vi "Wire Tag Terminals.vi"(6 "State":T1={"Worker Library Path"=path "", "Block Label"="", "Types"=[], "Selections"=[], "Icon"={"image type"=0, "image depth"=0, "image"=[], "mask"=[], "colors"=[], "Rectangle"={"left"=0, "top"=0, "right"=0, "bottom"=0}}, "Errors"={"Terminals"=[], "Generate"={"status"=FALSE, "code"=0, "source"=""}, "General"={"status"=FALSE, "code"=0, "source"=""}}, "Calculated Sizes"={"Block Width"=0, "Block Height"=0, "Half Width"=0, "Icon Top"=0, "Icon Bottom"=0, "Label Width"=0, "Half Label"=0, "Label Top"=0, "Text Width"=0, "Half Text"=0, "Text Height"=0, "Label Height"=0, "Expanded Width"=0, "Label Bottom"=0, "Expanded Top"=0, "Expanded Bottom"=0, "Expanded Height"=0, "Min Height"=0, "Max Height"=0}, "Special Terminal Indices"={"Action"=-1, "Init"=-1, "Tag"=-1, "State in"=-1, "State out"=-1, "Error"=-1}, "Terminals"=[]}, 8 "error in (no error)":errorcluster, 10 "Grouped Terms":T13, 11 "Refs In":T15) -> (0 "error out":errorcluster, 3 "Refs":T15)   [LabVIEW 2022 SP3, in "FlexBlocks Support.lvlib"]
uses:
  FlexBlocks Support.lvlib
  SM Refs.ctl
  Grouped Terms.ctl
  Terminal Group.ctl
  Type Descriptor.ctl
  Terminal Direction.ctl
  Value Mode.ctl
  Special Terminal.ctl
  Terminal State.ctl
  Flex Block/State.ctl
  <vilib>/picture/picture.llb/imagedata.ctl
  XNode Errors.ctl
  Calculated Sizes.ctl
  Special Terminal Indices.ctl
  Terminal Status.ctl
  Terminal Draw Style.ctl
  Flex Block/Flex Block.xnode
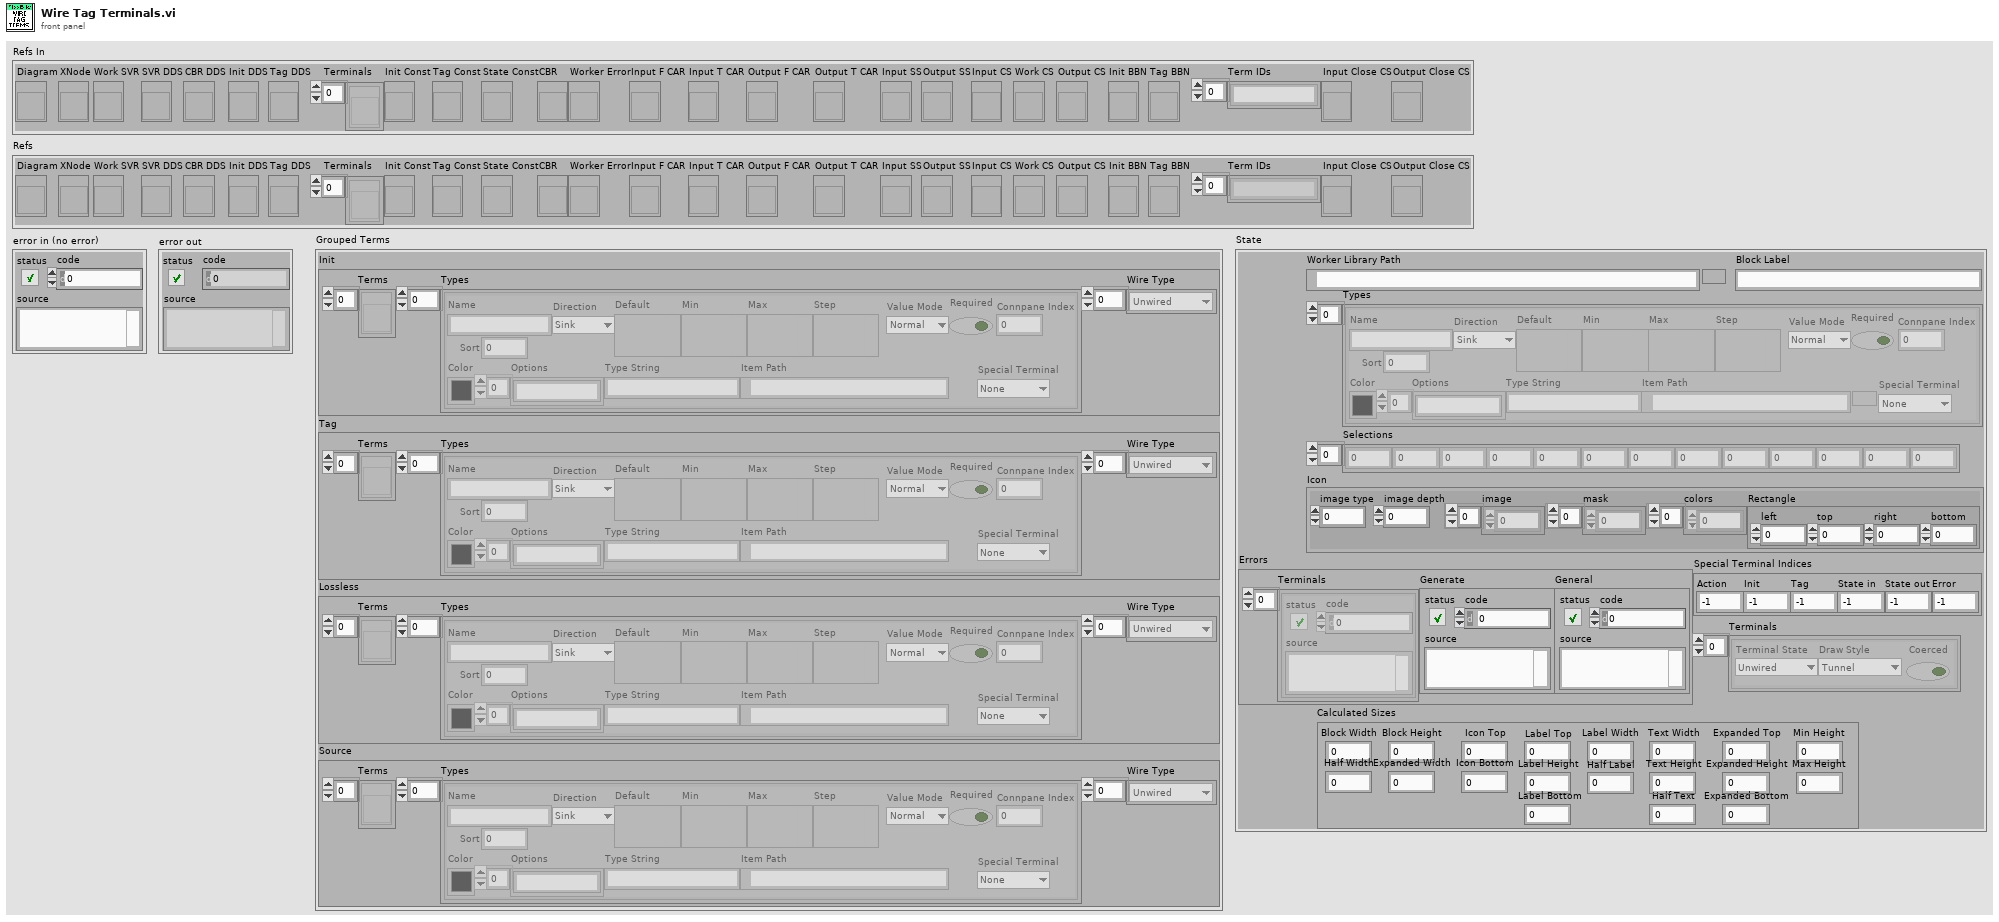
[diagram p1: front panel]
types:
  T1 = typedef "Flex Block.xnode/State.ctl" = cluster{"Worker Library Path":path, "Block Label":string, "Types":T2[], "Selections":i32[], "Icon":T6, "Errors":T7, "Calculated Sizes":T8, "Special Terminal Indices":T9, "Terminals":T10[]}
  T2 = typedef "FlexBlocks Support.lvlib/Type Descriptor.ctl" = cluster{"Name":string, "Direction":T3, "Default":variant, "Min":variant, "Max":variant, "Step":variant, "Value Mode":T4, "Color":u32, "Options":string[], "Type String":string, "Item Path":path, "Required":bool, "Connpane Index":i32, "Special Terminal":T5, "Sort":i32}
  T3 = typedef "FlexBlocks Support.lvlib/Terminal Direction.ctl" = enum16{"Sink", "Source"}
  T4 = typedef "FlexBlocks Support.lvlib/Value Mode.ctl" = enum16{"Normal", "Range", "Select"}
  T5 = typedef "FlexBlocks Support.lvlib/Special Terminal.ctl" = enum16{"None", "Action", "Init", "Tag", "State in", "State out", "Error"}
  T6 = typedef "imagedata.ctl" = cluster{"image type":i32, "image depth":i32, "image":u8[], "mask":u8[], "colors":u32[], "Rectangle":cluster{"left":i16, "top":i16, "right":i16, "bottom":i16}}
  T7 = typedef "FlexBlocks Support.lvlib/XNode Errors.ctl" = cluster{"Terminals":errorcluster[], "Generate":errorcluster, "General":errorcluster}
  T8 = typedef "FlexBlocks Support.lvlib/Calculated Sizes.ctl" = cluster{"Block Width":i32, "Block Height":i32, "Half Width":i32, "Icon Top":i32, "Icon Bottom":i32, "Label Width":i32, "Half Label":i32, "Label Top":i32, "Text Width":i32, "Half Text":i32, "Text Height":i32, "Label Height":i32, "Expanded Width":i32, "Label Bottom":i32, "Expanded Top":i32, "Expanded Bottom":i32, "Expanded Height":i32, "Min Height":i32, "Max Height":i32}
  T9 = typedef "FlexBlocks Support.lvlib/Special Terminal Indices.ctl" = cluster{"Action":i32, "Init":i32, "Tag":i32, "State in":i32, "State out":i32, "Error":i32}
  T10 = typedef "FlexBlocks Support.lvlib/Terminal Status.ctl" = cluster{"Terminal State":T11, "Draw Style":T12, "Coerced":bool}
  T11 = typedef "FlexBlocks Support.lvlib/Terminal State.ctl" = enum16{"Unwired", "BadType", "BadRef", "Channel", "Value", "Control Ref"}
  T12 = typedef "FlexBlocks Support.lvlib/Terminal Draw Style.ctl" = enum16{"Tunnel", "BadType", "BadRef", "Channel", "Value", "Control Ref"}
  T13 = typedef "FlexBlocks Support.lvlib/Grouped Terms.ctl" = cluster{"Init":T14, "Tag":T14, "Lossless":T14, "Source":T14}
  T14 = typedef "FlexBlocks Support.lvlib/Terminal Group.ctl" = cluster{"Terms":refnum<vi>[], "Types":T2[], "Wire Type":T11[]}
  T15 = typedef "FlexBlocks Support.lvlib/SM Refs.ctl" = cluster{"Diagram":refnum<vi>, "XNode":refnum<vi>, "Work SVR":refnum<vi>, "SVR DDS":refnum<vi>, "CBR DDS":refnum<vi>, "Init DDS":refnum<vi>, "Tag DDS":refnum<vi>, "Terminals":refnum<vi>[], "Init Const":refnum<vi>, "Tag Const":refnum<vi>, "State Const":refnum<vi>, "CBR":refnum<vi>, "Worker Error":refnum<vi>, "Input F CAR":refnum<vi>, "Input T CAR":refnum<vi>, "Output F CAR":refnum<vi>, "Output T CAR":refnum<vi>, "Input SS":refnum<vi>, "Output SS":refnum<vi>, "Input CS":refnum<vi>, "Work CS":refnum<vi>, "Output CS":refnum<vi>, "Init BBN":refnum<vi>, "Tag BBN":refnum<vi>, "Term IDs":string[], "Input Close CS":refnum<vi>, "Output Close CS":refnum<vi>}
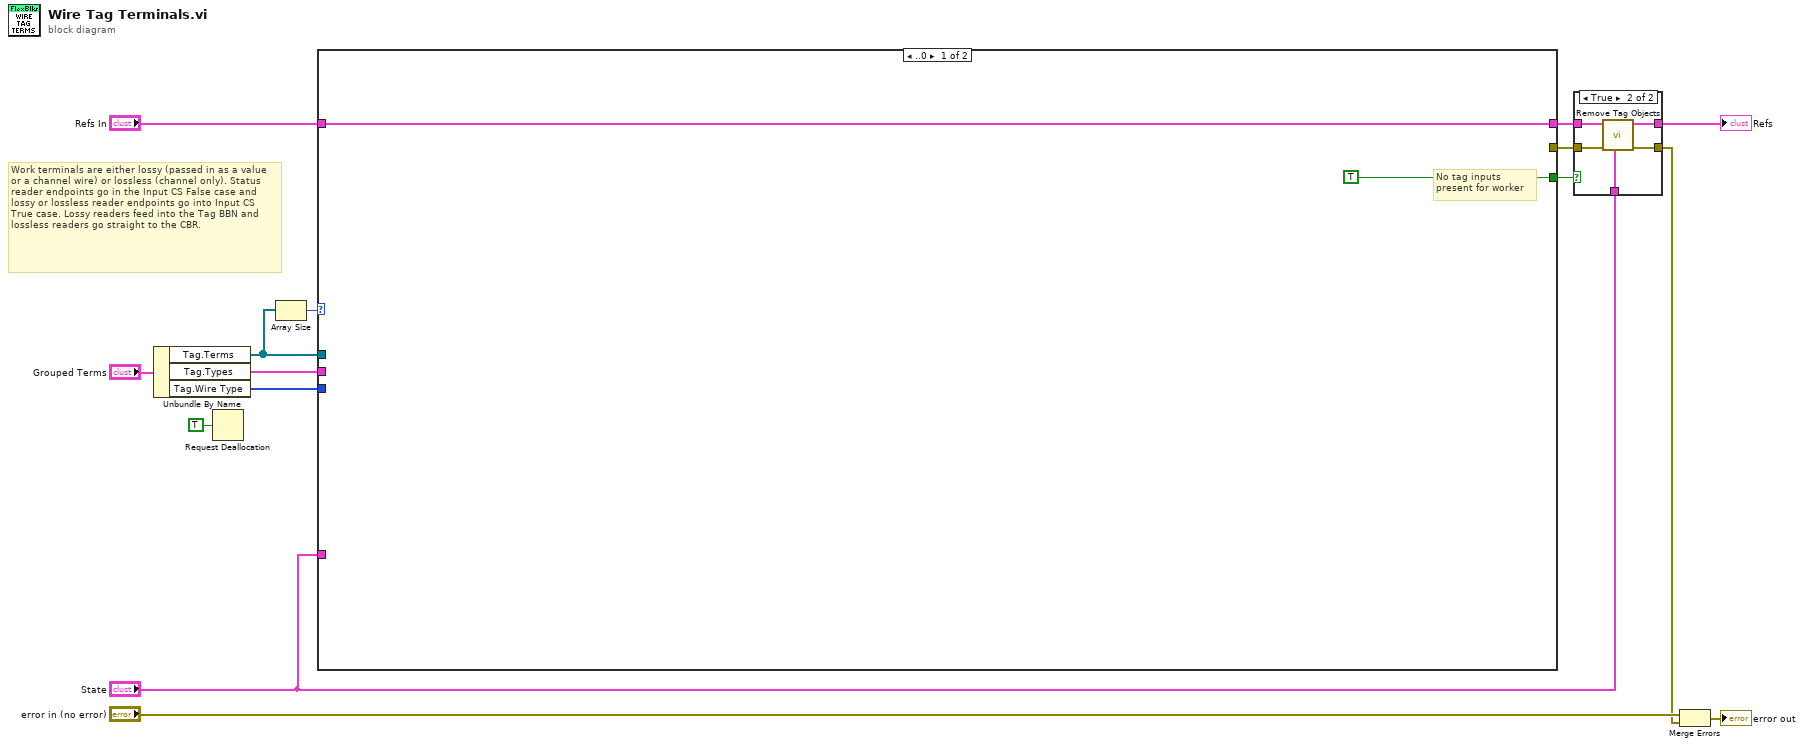
[diagram p0: block diagram]
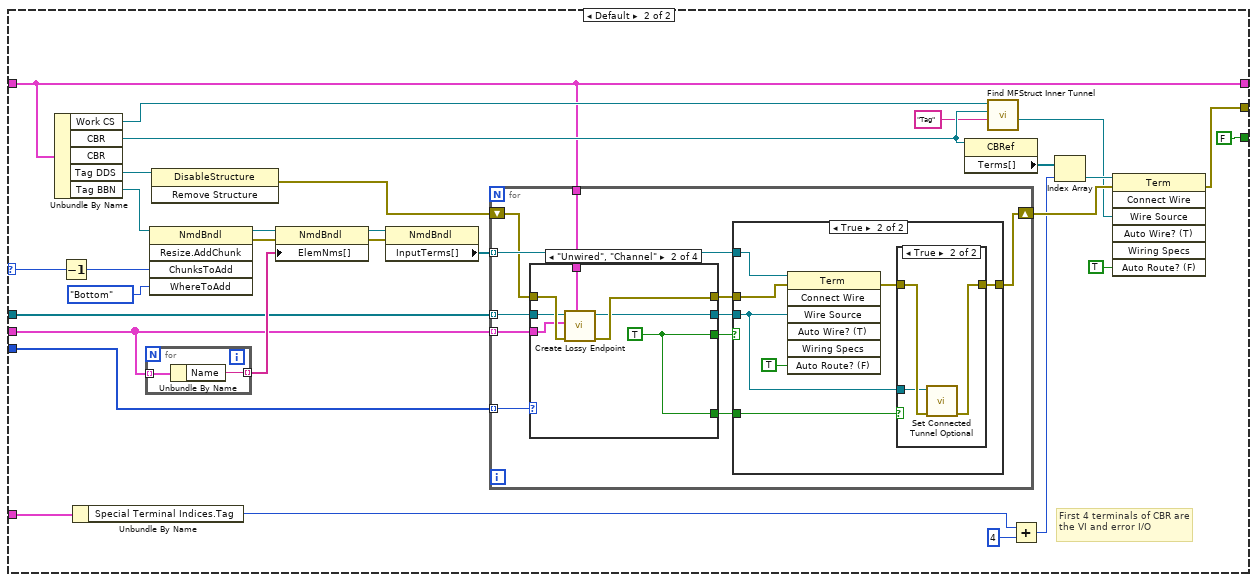
[diagram p2: hidden frame]
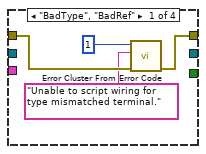
[diagram p3: hidden frame]
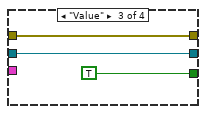
[diagram p4: hidden frame]
diagram:
  # "Work terminals are either lossy (passed in as a value or a channel wire) or lossless (channel only). Status reader endpoints go in the Input CS False case and lossy or lossless reader endpoints go into Input CS True case. Lossy readers feed into the Tag BBN and lossless readers go straight to the CBR."
  n1 = Unbundle By Name("Grouped Terms") -> ("Tag.Terms"=w13:refnum<vi>[], "Tag.Types"=w12:T2[], "Tag.Wire Type"=w3:T11[])
  n2 = Request Deallocation(TRUE ("flag")) -> ()
  n3 = Array Size(array=w13) -> (size(s)=w14:i32)
  n4 = case shown="..0" w14 {
    selector: w14 -> [_ w24]
    tunnel: w13 -> [_ w22]
    tunnel: w12 -> [_ w23]
    tunnel: "State" -> [_ w21]
    tunnel: "Refs In" -> [w17 w19]
    tunnel: [w17 w19] -> w10
    tunnel: [TRUE FALSE] -> w4
    tunnel: w3 -> [_ w20]
    tunnel: [_ w18] -> w1
    frame ..0 {
      # "No tag inputs present for worker"
    }
    frame Default {
      # "First 4 terminals of CBR are the VI and error I/O"
      n5 = Unbundle By Name(w19) -> ("Work CS"=w31:refnum<vi>, "CBR"=w30:refnum<vi>, "Tag DDS"=w44:refnum<vi>, "Tag BBN"=w43:refnum<vi>)  [unwired: 1 out]
      n6 = Decrement(x=w24) -> (x-1=w42:i32)
      n7 = Unbundle By Name(w21) -> ("Special Terminal Indices.Tag"=w33:i32)
      n8 = for {
        tunnel: w23 -> [w49] mode=indexing
        tunnel: [w48] -> w37 mode=indexing
        n9 = Unbundle By Name(w49) -> ("Name"=w48:string)
      }
      n10 = invoke class="NmdBndl" method="Resize.AddChunk"(reference=w43, "ChunksToAdd"=w42, "WhereToAdd"=enum8{"Bottom", "Top"}."Bottom" ("Where To Add")) -> (reference out=w39:refnum<vi>, error out=w38:errorcluster)  [unwired: 2 in, 3 out]
      n11 = invoke class="DisableStructure" method="Remove Structure"(reference=w44) -> (error out=w45:errorcluster)  [unwired: 2 in, 2 out]
      n12 = property class="NmdBndl"(reference=w39, error in=w38, "ElemNms[]"=w37) -> (reference out=w40:refnum<vi>, error out=w35:errorcluster)
      n13 = property class="NmdBndl"(reference=w40, error in=w35) -> ("InputTerms[]"=w36:refnum<vi>[])  [unwired: 2 out]
      n14 = for {
        tunnel: w22 -> [w57] mode=indexing
        tunnel: w23 -> [w56] mode=indexing
        tunnel: w36 -> [w60] mode=indexing
        shift-right: [w59] -> w46
        shift-left: w45 -> [w53]
        tunnel: w20 -> [w58] mode=indexing
        tunnel: w19 -> [w51]
        n15 = case shown="\"Unwired\", \"Channel\"" w58 {
          tunnel: w57 -> [_ w69 w73 _]
          tunnel: w56 -> [_ w68 _ _]
          tunnel: [_ w65 TRUE _] -> w55
          tunnel: [_ w67 w73 _] -> w54
          tunnel: w53 -> [w64 w70 w72 w75]
          tunnel: [w63 w71 w72 w75] -> w52
          tunnel: w51 -> [_ w66 _ _]
          tunnel: [_ w65 _ _] -> w50
          frame "BadType", "BadRef" {
            n16 = call <vilib>:"Error Cluster From Error Code.vi"("error in (no error)"=w64, "error message (\"\")"="Unable to script wiring for type mismatched terminal." ("error message (\"\")"), "error code (0)"=1) -> ("error out"=w63:errorcluster)  [unwired: 6 in]
          }
          frame "Unwired", "Channel" {
            w65 = TRUE
            n17 = call "Create Lossy Endpoint.vi"("Refs"=w66, "error in (no error)"=w70, "Type Descriptor"=w68, "Channel Term"=w69) -> ("error out"=w71:errorcluster, "Element Term"=w67:refnum<vi>)  [unwired: 6 in]
          }
          frame "Value" {
          }
          frame "Control Ref" {
          }
        }
        n18 = case shown="True" w55 {
          tunnel: w60 -> [_ w83]
          tunnel: [w76 w78] -> w59
          tunnel: w54 -> [_ w77]
          tunnel: w52 -> [w76 w81]
          tunnel: w50 -> [_ w80]
          frame False {
          }
          frame True {
            n19 = invoke class="Term" method="Connect Wire"(reference=w83, error in=w81, "Wire Source"=w77, "Auto Route? (F)"=TRUE) -> (error out=w79:errorcluster)  [unwired: 3 in, 6 out]
            n20 = case shown="True" w80 {
              tunnel: w79 -> [w84 w87]
              tunnel: [w84 w85] -> w78
              tunnel: w77 -> [_ w86]
              frame False {
              }
              frame True {
                n21 = call "Set Connected Tunnel Optional.vi"("error in (no error)"=w87, "Term Refnum"=w86) -> ("error out"=w85:errorcluster)  [unwired: 9 in]
              }
            }
          }
        }
      }
      n22 = property class="CBRef"(reference=w30) -> ("Terms[]"=w34:refnum<vi>[])  [unwired: 1 in, 2 out]
      n23 = call "Find MFStruct Inner Tunnel.vi"("Tunnel Name"="Tag", "Contained GObject"=w30, "MFStruct"=w31) -> ("Inside Tunnel"=w26:refnum<vi>)  [unwired: 5 in, 3 out]
      n24 = Add(x=w33, y=4) -> (x+y=w28:i32)
      n25 = Index Array(array=w34, index=w28) -> (element=w27:refnum<vi>)
      n26 = invoke class="Term" method="Connect Wire"(reference=w27, error in=w46, "Wire Source"=w26, "Auto Route? (F)"=TRUE) -> (error out=w18:errorcluster)  [unwired: 3 in, 6 out]
    }
  }
  n27 = case shown="True" w4 {
    tunnel: w10 -> [w89 w94]
    tunnel: [w89 w93] -> w9
    tunnel: "State" -> [_ w92]
    tunnel: [w88 w91] -> w5
    tunnel: w1 -> [w88 w90]
    frame False {
    }
    frame True {
      n28 = call "Remove Tag Objects.vi"("State"=w92, "error in (no error)"=w90, "Refs In"=w94) -> ("error out"=w91:errorcluster, "Refs"=w93:T15)  [unwired: 7 in]
    }
  }
  "Refs" <- w9
  n29 = Merge Errors("error in (no error)", w5) -> (→"error out":errorcluster)
